vi "AddManyToQueue.vi"(9 "Cmds":string, 11 "Queue in":refnum<queue>) -> (3 "Queue out":refnum<queue>)   [LabVIEW 2017]
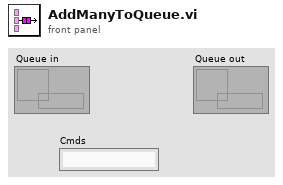
[diagram p1: front panel]
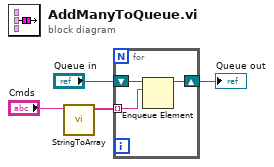
[diagram p0: block diagram]
diagram:
  n1 = call <userlib>:"StringToArray.vi"("write buffer"="Cmds") -> ("Array"=w1:string[])  [unwired: 10 in]
  n2 = for {
    shift-right: [w7] -> w3
    shift-left: "Queue in" -> [w6]
    tunnel: w1 -> [w5] mode=indexing
    n3 = Enqueue Element(queue=w6, element=w5) -> (queue out=w7:refnum<queue>)  [unwired: 2 in, 2 out]
  }
  "Queue out" <- w3
